vi "subImagesAndBfiled.vi"(9 "B [T]":dbl, 11 "MagAnalysis_Online in":refnum<class "MagAnalysis_Online.lvclass">) -> (0 "image ok":bool[](array[boolean]), 1 "B[T]":dbl, 2 "new ROI":bool, 3 "MagAnalysis_Online out":refnum<class "MagAnalysis_Online.lvclass">, 4 "Numeric 2":u32, 5 "OK":bool[](array[boolean]))   [LabVIEW 2020, in "MagAnalysis_Online.lvclass"]
uses:
  MagAnalysis_Online.lvclass
  MagAnalysis_Online.lvclass/MagAnalysis_Online.ctl
panel:
  out "ROI 2":i32[][](array[numeric])
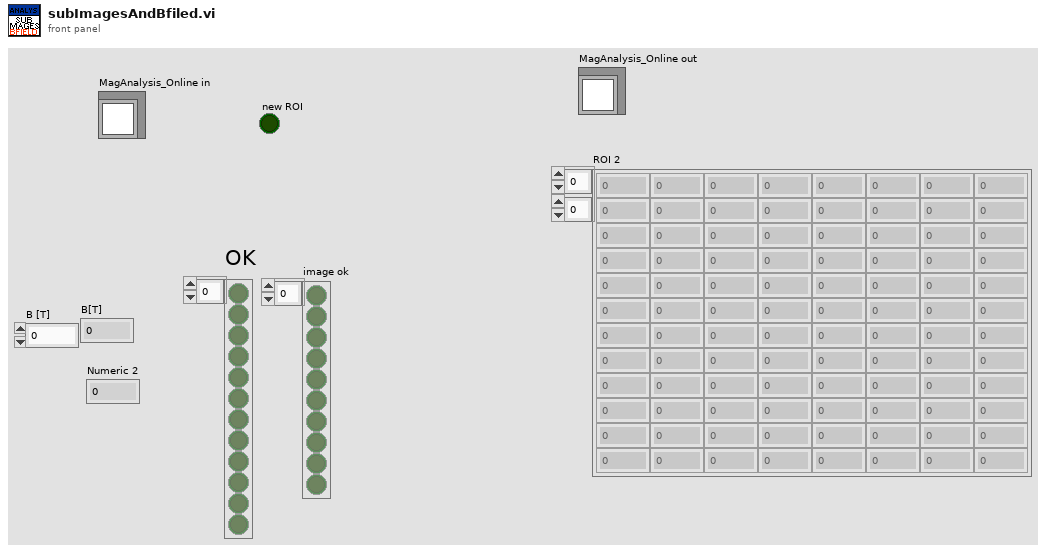
[diagram p1: front panel]
types:
  T1 = typedef "CamSettings_Typdef.ctl" = cluster{"Cam 0":T2, "Cam 1":T2, "Cam 2":T2, "Cam 3":T2}
  T2 = typedef "CamSettingSUB_TypDEf.ctl" = cluster{"position":dbl, "pixelsize":dbl, "start":dbl, "end":dbl, "center":dbl, "Lens":T3, "Forward":T4, "Spec_Calib_file 2":path, "map":path, "y size":i32, "UserROI":T5, "CamMaxPixel":cluster{"X":i32, "Y":i32}, "CamROI":T7}
  T3 = typedef "CamAndObj_TypDEf.ctl" = enum16{"FL1-f8x08", "FL1-f8x06", "FL1-f8", "ch300-f50", "FL2G-f8", "FL3M14-f8", "FL3M14-f8x08", "FL3M14-f8x08(2x2)"}
  T4 = typedef "OnOffTypeDef.ctl" = enum16{"off", "on"}
  T5 = typedef "userROI.ctl" = cluster{"Width":T6, "Hight":T6, "OffsetX":T6, "OffsetY":T6}
  T6 = typedef "BaseDriver.lvclass/numericVariable_TypeDef.ctl" = cluster{"Value":dbl, "Min":dbl, "Max":dbl, "StepSize":dbl, "Tolerance":dbl, "ValueActual":dbl}
  T7 = typedef "CamRoiTypDef.ctl" = cluster{"Width":dbl, "Hight":dbl, "OffsetX":dbl, "OffsetY":dbl}
  T8 = typedef "SubscriberCluster_TypDEf.ctl" = cluster{"tcp data event":T9, "Event Registration Refnum":refnum<event-registration>, "data queue":refnum<queue>, "Devices":string[], "Alias":string[], "Variable header":string[], "Devices ALL":string[]}
  T9 = typedef "tcp_new_data_event.ctl" = refnum<user-event>
  T10 = typedef "MagAnalysis_Online.lvclass/analysis_data_typdef.ctl" = cluster{"cam0":T11, "cam1":T11, "cam2":T11, "cam3":T11}
  T11 = typedef "IMAQ Image.ctl" = refnum<image>
  T12 = typedef "ROIStartfromCam_typdef.ctl" = cluster{"Cam0":T13, "Cam1":T13, "Cam2":T13, "Cam3":T13}
  T13 = typedef "classicROI_typDef.ctl" = cluster{"Width":dbl, "Hight":dbl, "OffsetX":dbl, "OffsetY":dbl}
  T14 = typedef "bgImages_tyudef.ctl" = cluster{"cam 0":T11, "cam 1":T11, "cam 2":T11, "cam 3":T11}
  T15 = typedef "dataTypdef.ctl" = cluster{"cam0":T11, "cam1":T11, "cam2":T11, "cam3":T11, "Bfield":dbl, "ROI":T12}
  T16 = cluster{"[0]":T11, "[1]":T11, "[2]":T11, "[3]":T11}
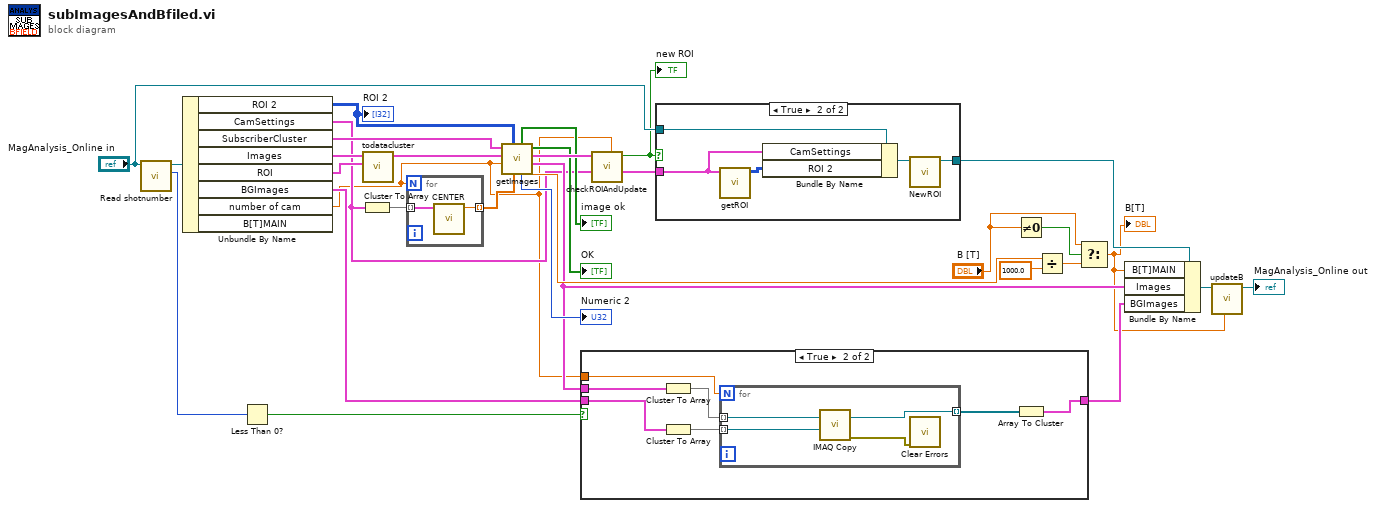
[diagram p0: block diagram]
diagram:
  n1 = call-dynamic "Read shotnumber.vi"("BaseDriver in"="MagAnalysis_Online in") -> ("shotnumber"=w21:i32, "BaseDriver out"=w20:refnum<class "MagAnalysis_Online.lvclass">)  [unwired: 7 in, 2 out]
  n2 = Unbundle By Name(w20) -> ("ROI 2"=w12:i32[][], "CamSettings"=w6:T1, "SubscriberCluster"=w31:T8, "Images"=w28:T10, "ROI"=w29:T12, "BGImages"=w17:T14, "number of cam"=w3:dbl)  [unwired: 1 out]
  "ROI 2" <- w12
  n3 = Less Than 0?(x=w21) -> (x < 0?=w19:bool)
  n4 = Cluster To Array(cluster=w6) -> (array=w7:T2[])
  n5 = call "todatacluster.vi"("ROI"=w29, "Images"=w28) -> ("data"=w30:T15)  [unwired: 9 in]
  n6 = for {
    N: w3 -> [_]
    tunnel: w7 -> [w33] mode=indexing
    tunnel: [w32] -> w5 mode=indexing
    n7 = call "CENTER.vi"("Cam 0"=w33) -> ("Numeric"=w32:dbl)  [unwired: 10 in]
  }
  n8 = call "getImages.vi"("Array"=w5, "ROI 2"=w12, "number of cam"=w3, "data"=w30, "SubscriberCluster"=w31) -> ("B[mT]"=w26:dbl, "Images"=w11:T10, "ROI"=w24:T12, "OK"=→"OK":bool[], "Numeric"=→"Numeric 2":u32, "image ok"=→"image ok":bool[])  [unwired: 1 in]
  n9 = case shown="True" w19 {
    tunnel: w11 -> [_ w41]
    tunnel: [w34 w36] -> w18
    tunnel: w17 -> [w34 w40]
    tunnel: w3 -> [_ w35]
    frame False {
    }
    frame True {
      n10 = Cluster To Array(cluster=w41) -> (array=w38:T11[])
      n11 = Cluster To Array(cluster=w40) -> (array=w39:T11[])
      n12 = for {
        N: w35 -> [_]
        tunnel: w39 -> [w45] mode=indexing
        tunnel: w38 -> [w44] mode=indexing
        tunnel: [w43] -> w37 mode=indexing
        n13 = call "IMAQ Copy"("Image Dst"=w45, "Image Src"=w44) -> ("error out"=w42:errorcluster, "Image Dst Out"=w43:T11)  [unwired: 4 in]
        n14 = call <vilib>:"Clear Errors.vi"("error in (no error)"=w42) -> ()  [unwired: 5 in, 2 out]
      }
      n15 = Array To Cluster(array=w37) -> (cluster=w36:T16)
    }
  }
  n16 = call "checkROIAndUpdate.vi"("Settings.number of cam"=w3, "Settings.CamSettings 3"=w6, "ROI in"=w24) -> ("Settings.CamSettings 2"=w4:T1, "new ROI"=w9:bool)  [unwired: 7 in]
  "new ROI" <- w9
  n17 = case shown="True" w9 {
    tunnel: "MagAnalysis_Online in" -> [w46 w51]
    tunnel: [w46 w49] -> w27
    tunnel: w4 -> [_ w48]
    frame False {
    }
    frame True {
      n18 = call "getROI.vi"("CamSettings"=w48) -> ("ROI"=w47:i32[][])  [unwired: 10 in]
      n19 = Bundle By Name(cluster=w51, "CamSettings"=w48, "ROI 2"=w47) -> (w50:refnum<class "MagAnalysis_Online.lvclass">)
      n20 = call "NewROI.vi"("MagAnalysis_Online in"=w50) -> ("MagAnalysis_Online out"=w49:refnum<class "MagAnalysis_Online.lvclass">)  [unwired: 10 in]
    }
  }
  n21 = Not Equal To 0?(x="B [T]") -> (x != 0?=w15:bool)
  n22 = Divide(x=w26, y=1000.0) -> (x/y=w13:dbl)
  n23 = Select(t="B [T]", s=w15, f=w13) -> (s? t:f=w2:dbl)
  "B[T]" <- w2
  n24 = Bundle By Name(cluster=w27, "B[T]MAIN"=w2, "Images"=w11, "BGImages"=w18) -> (w8:refnum<class "MagAnalysis_Online.lvclass">)
  n25 = call "updateB.vi"("B [T] new"=w2, "MagAnalysis_Online in"=w8) -> ("MagAnalysis_Online out"=→"MagAnalysis_Online out":refnum<class "MagAnalysis_Online.lvclass">)  [unwired: 9 in]
